vi "Add NI-SWITCH Custom Device.vi"(8 "error in":errorcluster, 10 "name":string="NI-SWITCH", 11 "target in":refnum<k24>) -> (0 "error out":errorcluster, 2 "ni-switch custom device":T1 format="%.0x", 3 "target out":refnum<k24>)   [LabVIEW 2020, in "NI-SWITCH Scripting.lvlib"]
doc: "Creates and adds a new instance of the NI-SWITCH custom device to the specified target."
uses:
  NI-SWITCH Scripting.lvlib
  <vilib>/NI VeriStand/Custom Device API/Custom Device Item Ref.ctl
  NationalInstruments.VeriStand.SystemDefinitionAPI
  Shared/Constants.vi
  Shared/NI-SWITCH Shared.lvlib
  <vilib>/NI VeriStand/Custom Device Tools/Custom Device Utility Library/Custom Device Utility Library.lvlib
  <vilib>/NI VeriStand/Custom Device API/Custom Device API.lvlib
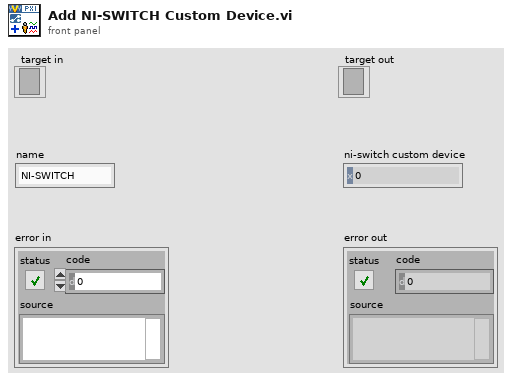
[diagram p1: front panel]
types:
  T1 = typedef "Custom Device API.lvlib/Custom Device Item Ref.ctl" = u64
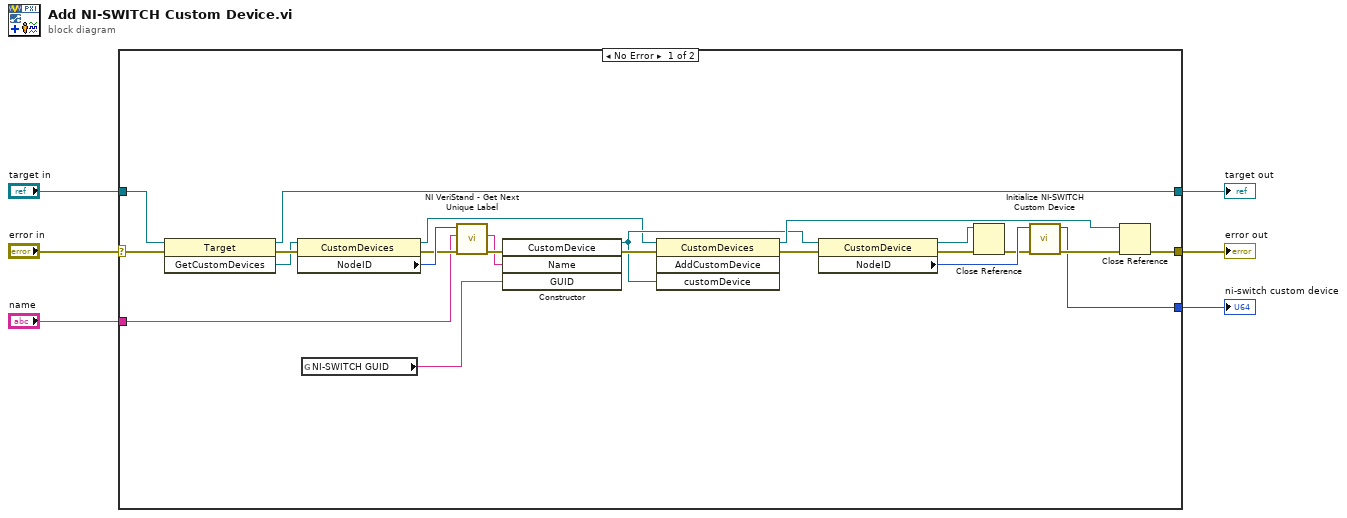
[diagram p0: block diagram]
diagram:
  n1 = case shown="No Error" "error in" {
    selector: "error in" -> [w26 w31]
    tunnel: "target in" -> [w25 w30]
    tunnel: [w24 w30] -> w2
    tunnel: [w21 w31] -> w6
    tunnel: [w22 _] -> w4
    tunnel: "name" -> [w7 _]
    frame No Error {
      n2 = invoke class="Target" method="GetCustomDevices"(reference=w25, error in=w26) -> (reference out=w24:refnum<k24>, error out=w29:errorcluster, "GetCustomDevices"=w13:refnum<k24>)  [unwired: 1 in]
      n3 = property class="CustomDevices"(reference=w13, error in=w29) -> (reference out=w10:refnum<k24>, error out=w11:errorcluster, "NodeID"=w12:u64)
      n4 = global read "Constants.vi" "NI-SWITCH GUID"() -> (w23:string)
      n5 = call <vilib>:"NI VeriStand - Get Next Unique Label.vi"("error in (no error)"=w11, "Label"=w7, "Parent Ref in"=w12) -> ("error out"=w9:errorcluster, "Label out"=w8:string)  [unwired: 5 in, 2 out]
      n6 = constructor class="CustomDevice"(error in=w9, "Name"=w8, "GUID"=w23) -> (reference out=w14:refnum<k24>, error out=w20:errorcluster)  [unwired: 2 in, 3 out]
      n7 = invoke class="CustomDevices" method="AddCustomDevice"(reference=w10, error in=w20, "customDevice"=w14) -> (reference out=w28:refnum<k24>, error out=w19:errorcluster)  [unwired: 1 in, 2 out]
      n8 = property class="CustomDevice"(reference=w14, error in=w19) -> (reference out=w17:refnum<k24>, error out=w16:errorcluster, "NodeID"=w18:u64)
      n9 = Close Reference(reference=w17, error in (no error)=w16) -> (error out=w15:errorcluster)
      n10 = call "Initialize NI-SWITCH Custom Device.vi"("error in"=w15, "ni-switch custom device in"=w18) -> ("error out"=w27:errorcluster, "ni-switch custom device out"=w22:T1)  [unwired: 7 in, 1 out]
      n11 = Close Reference(reference=w28, error in (no error)=w27) -> (error out=w21:errorcluster)
    }
    frame Error {
    }
  }
  "error out" <- w6
  "ni-switch custom device" <- w4
  "target out" <- w2
